vi "newIDfinder.vi"(10 "dup Data":T1[](array[typedef])) -> (2 "ID":u32)   [LabVIEW 2014, in "Contact Data.lvlib"]
uses:
  Contact Data.lvlib
  Contact.ctl
  Position.ctl
  Controls.ctl
  DestinationCluster.ctl
  DesinationControls.ctl
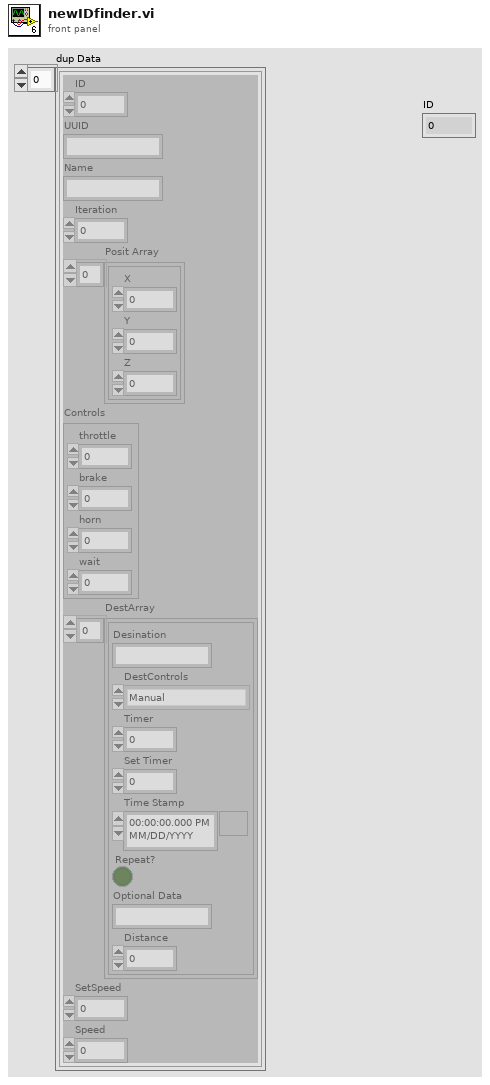
[diagram p1: front panel]
types:
  T1 = typedef "Contact Data.lvlib/Contact.ctl" = cluster{"ID":u32, "UUID":string, "Name":string, "Iteration":i32, "Posit Array":T2[], "Controls":T3, "DestArray":T4[], "SetSpeed":dbl, "Speed":dbl}
  T2 = typedef "Contact Data.lvlib/Position.ctl" = cluster{"X":dbl, "Y":dbl, "Z":dbl}
  T3 = typedef "Contact Data.lvlib/Controls.ctl" = cluster{"throttle":dbl, "brake":dbl, "horn":dbl, "wait":dbl}
  T4 = typedef "Contact Data.lvlib/DestinationCluster.ctl" = cluster{"Desination":string, "DestControls":T5, "Timer":u32, "Set Timer":u32, "Time Stamp":timestamp, "Repeat?":bool, "Optional Data":string, "Distance":dbl}
  T5 = typedef "Contact Data.lvlib/DesinationControls.ctl" = enum16{"Tracker", "Manual", "Stop", "Station DateTime", "Station Timer", "Maintain"}
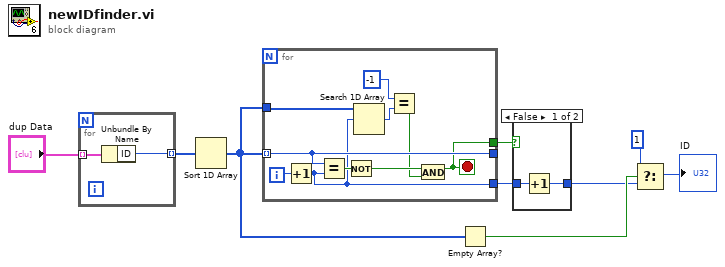
[diagram p0: block diagram]
diagram:
  n1 = for {
    tunnel: "dup Data" -> [w11] mode=indexing
    tunnel: [w10] -> w8 mode=indexing
    n2 = Unbundle By Name(w11) -> ("ID"=w10:u32)
  }
  n3 = Sort 1D Array(array=w8) -> (sorted array=w4:u32[])
  n4 = for {
    tunnel: w4 -> [w21] mode=indexing
    tunnel: [w21] -> _
    tunnel: [w13] -> w1
    tunnel: [w16] -> w3
    tunnel: w4 -> [w17]
    i -> [w20]
    stop <- w13 stop-if-true
    n5 = Increment(x=w20) -> (x+1=w16:i32)
    n6 = Equal?(x=w21, y=w16) -> (x = y?=w19:bool)
    n7 = Not(x=w19) -> (.not. x?=w18:bool)
    n8 = Search 1D Array(1D array=w17, element=w16) -> (index of element=w15:i32)  [unwired: 1 in]
    n9 = Equal?(x=-1 ("x+1"), y=w15) -> (x = y?=w12:bool)
    n10 = And(x=w18, y=w12) -> (x .and. y?=w13:bool)
  }
  n11 = Empty Array?(array=w4) -> (empty?=w7:bool)
  n12 = case shown="False" w1 {
    tunnel: w3 -> [w23 w24]
    tunnel: [w22 w24] -> w2
    frame False {
      n13 = Increment(x=w23) -> (x+1=w22:i32)
    }
    frame True {
    }
  }
  n14 = Select(t=u32 1, s=w7, f=w2) -> (s? t:f=→"ID":u32)
